vi "RtdeGetState.vi"(8 "Rtde":refnum<k24>, 11 "error in":errorcluster) -> (0 "State":T1 {"State" items=["Disabled", "Connecting", "Started", "Paused"]}, 1 "Connected":bool, 3 "error out":errorcluster)   [LabVIEW 2023, in "UnderAutomation.UniversalRobots.lvlib"]
uses:
  UnderAutomation.UniversalRobots.lvlib
  C:/Users/fg/Documents/UniversalRobots.vi/UnderAutomation.UniversalRobots/lib/UnderAutomation.UniversalRobots.dll
  lib/UnderAutomation.UniversalRobots.dll
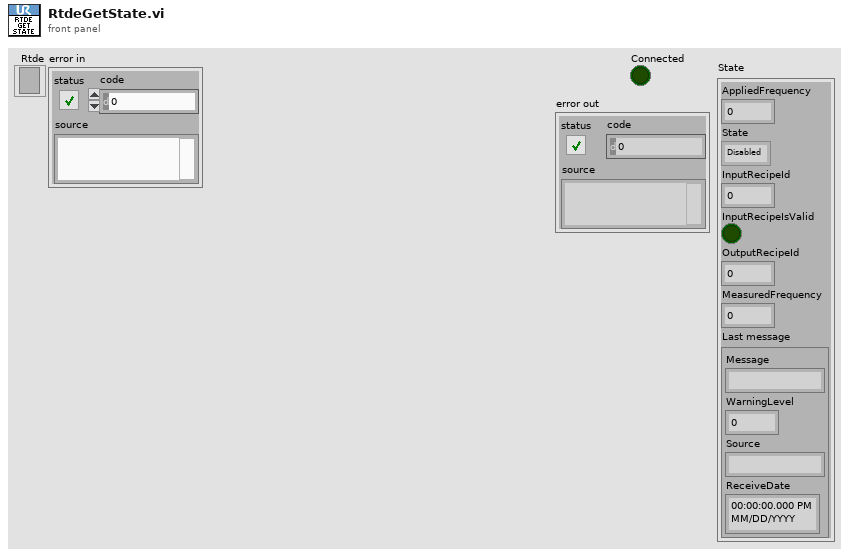
[diagram p1: front panel]
types:
  T1 = cluster{"AppliedFrequency":dbl, "State":i32, "InputRecipeId":u8, "InputRecipeIsValid":bool, "OutputRecipeId":u8, "MeasuredFrequency":dbl, "Last message":cluster{"Message":string, "WarningLevel":u8, "Source":string, "ReceiveDate":timestamp}}
  T2 = cluster{"Message":string, "WarningLevel":u8, "Source":string, "ReceiveDate":timestamp}
  T3 = cluster{"AppliedFrequency":dbl, "State":i32, "InputRecipeId":u8, "InputRecipeIsValid":bool, "OutputRecipeId":u8, "MeasuredFrequency":dbl, cluster{"Message":string, "WarningLevel":u8, "Source":string, "ReceiveDate":timestamp}}
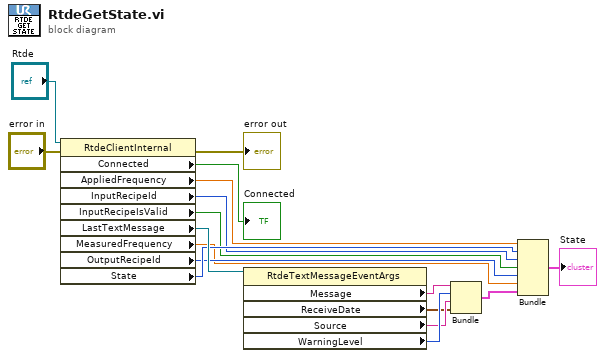
[diagram p0: block diagram]
diagram:
  n1 = property class="RtdeClientInternal"(reference="Rtde", error in="error in") -> (error out=→"error out":errorcluster, "Connected"=→"Connected":bool, "AppliedFrequency"=w7:dbl, "InputRecipeId"=w5:u8, "InputRecipeIsValid"=w4:bool, "LastTextMessage"=w13:refnum<k24>, "MeasuredFrequency"=w2:dbl, "OutputRecipeId"=w3:u8, "State"=w6:i32)  [unwired: 1 out]
  n2 = property class="RtdeTextMessageEventArgs"(reference=w13) -> ("Message"=w12:string, "ReceiveDate"=w9:timestamp, "Source"=w10:string, "WarningLevel"=w11:u8)  [unwired: 1 in, 2 out]
  n3 = Bundle("Message"=w12, "WarningLevel"=w11, "Source"=w10, "ReceiveDate"=w9) -> (w1:T2)  [unwired: 1 in]
  n4 = Bundle("AppliedFrequency"=w7, "State"=w6, "InputRecipeId"=w5, "InputRecipeIsValid"=w4, "OutputRecipeId"=w3, "MeasuredFrequency"=w2, w1) -> (→"State":T3)  [unwired: 1 in]
